vi "test_shuffle_string.vi"() -> ()   [LabVIEW 2021]
uses:
  4a7fb05e-3d81-3fec-48d6-f350c2acd13f.vi
  4a7fb05e-3d81-3fec-48d6-f350c2acd13f.vi/583681f2-f74d-3fed-28b4-9e1d217ae73f.vi
panel:
  out "shuffled array":string
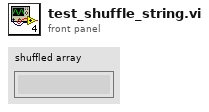
[diagram p1: front panel]
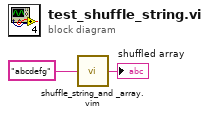
[diagram p0: block diagram]
diagram:
  n1 = call "shuffle_string_and _array.vim"("array"="abcdefg") -> ("shuffled array"=→"shuffled array":string)
